vi "Gyro Turn.vi"(6 "degrees":dbl, 9 "If right":bool, 10 "GyroDevRef":T7 {"Sample Rate" min=0.25 max=100.0 step=0.25}, 11 "RobotDriveDevRef in":T1) -> (3 "RobotDriveDevRef out":T1)   [LabVIEW 2017]
uses:
  <vilib>/Rock Robotics/WPI/RobotDrive/WPI_RobotDriveDevRef.ctl
  <vilib>/Rock Robotics/WPI/MotorControl/WPI_MotorControlDeviceRef.ctl
  <vilib>/Rock Robotics/WPI/MotorControl/WPI_MotorControlType.ctl
  <vilib>/Rock Robotics/SystemInterfaces/DIO/FPGA_DIOPWMChannel.ctl
  <vilib>/Rock Robotics/WPI/PWM/WPI_PWMDeadband.ctl
  <vilib>/Rock Robotics/SystemInterfaces/DIO/FPGA_DIOChannel.ctl
  <vilib>/Rock Robotics/WPI/Gyro/WPI_GyroDevRef.ctl
  <vilib>/Rock Robotics/SystemInterfaces/AI/FPGA_AIChannel.ctl
  <vilib>/Rock Robotics/SystemInterfaces/spilib/spi_bus.ctl
  <vilib>/Rock Robotics/WPI/SafetyOutput/WPI_SafetyOutputConfigMenu.ctl
panel:
  # "Analog"
  # "XRS"
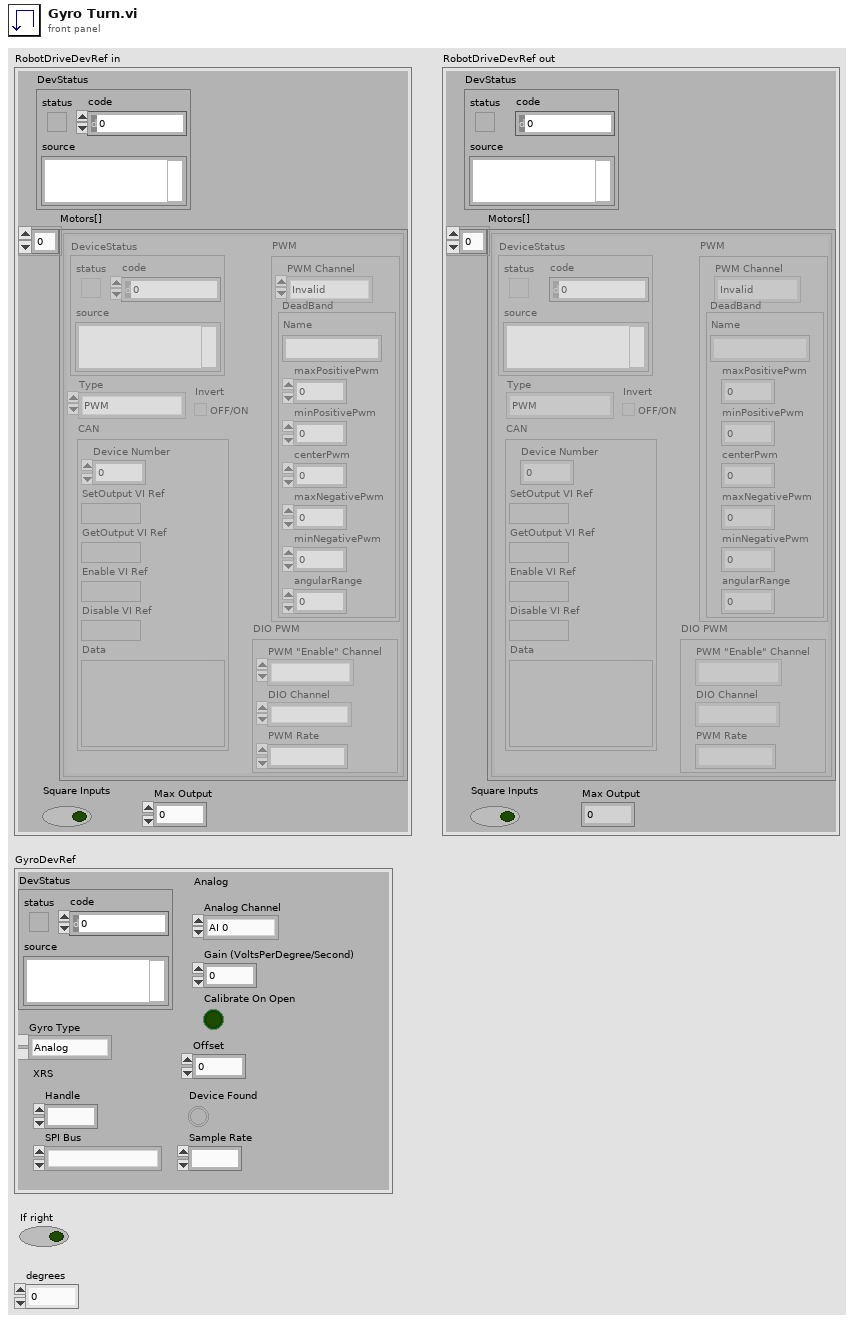
[diagram p1: front panel]
types:
  T1 = typedef "WPI_RobotDriveDevRef.ctl" = cluster{"DevStatus":errorcluster, "Motors[]":T2[], "Square Inputs":bool, "Max Output":dbl}
  T2 = typedef "WPI_MotorControlDeviceRef.ctl" = cluster{"DeviceStatus":errorcluster, "Type":T3, "PWM":cluster{"PWM Channel":T4, "DeadBand":T5}, "CAN":cluster{"Device Number":u8, "SetOutput VI Ref":variant, "GetOutput VI Ref":variant, "Enable VI Ref":variant, "Disable VI Ref":variant, "Data":variant}, "Invert":bool, "DIO PWM":cluster{"PWM \"Enable\" Channel":T4, "DIOChannel":T6, "PWM Rate":dbl}}
  T3 = typedef "WPI_MotorControlType.ctl" = enum16{"PWM", "CAN", "DIO PWM"}
  T4 = typedef "FPGA_DIOPWMChannel.ctl" = enum8{"PWM 0", "PWM 1", "PWM 2", "PWM 3", "PWM 4", "PWM 5", "PWM 6", "PWM 7", "PWM 8", "PWM 9", "PWM MXP 0", "PWM MXP 1", "PWM MXP 2", "PWM MXP 3", "PWM MXP 4", "PWM MXP 5", "PWM MXP 6", "PWM MXP 7", "PWM MXP 8", "PWM MXP 9", "Invalid"}
  T5 = typedef "WPI_PWMDeadband.ctl" = cluster{"Name":string, "maxPositivePwm":i32, "minPositivePwm":i32, "centerPwm":i32, "maxNegativePwm":i32, "minNegativePwm":i32, "angularRange":u16}
  T6 = typedef "FPGA_DIOChannel.ctl" = enum8{"DIO 0", "DIO 1", "DIO 2", "DIO 3", "DIO 4", "DIO 5", "DIO 6", "DIO 7", "DIO 8", "DIO 9", "DIO MXP 0", "DIO MXP 1", "DIO MXP 2", "DIO MXP 3", "DIO MXP 4", "DIO MXP 5", "DIO MXP 6", "DIO MXP 7", "DIO MXP 8", "DIO MXP 9", "DIO MXP 10", "DIO MXP 11", "DIO MXP 12", "DIO MXP 13", "DIO MXP 14", "DIO MXP 15", "SPI Port CS1", "SPI Port CS2", "SPI Port CS3", "SPI Port MISO", "SPI Port MOSI", "Invalid"}
  T7 = typedef "WPI_GyroDevRef.ctl" = cluster{"DevStatus":errorcluster, "Analog Channel":T8, "Gain (VoltsPerDegree/Second)":dbl, "Gyro Type":enum16{"Analog", "XRS450"}, "Handle":i32, "SPI Bus":T9, "Device Found":bool, "Sample Rate":dbl, "Calibrate On Open":bool, "Offset":dbl}
  T8 = typedef "FPGA_AIChannel.ctl" = enum8{"AI 0", "AI 1", "AI 2", "AI 3", "AI MXP 0", "AI MXP 1", "AI MXP 2", "AI MXP 3", "Invalid"}
  T9 = typedef "spi_bus.ctl" = enum16{"SPI On-Board, CS0", "SPI On-Board, CS1", "SPI On-Board, CS2", "SPI On-Board, CS3", "SPI MXP", "Invalid"}
  T10 = typedef "WPI_SafetyOutputConfigMenu.ctl" = enum16{"Enable", "Disable"}
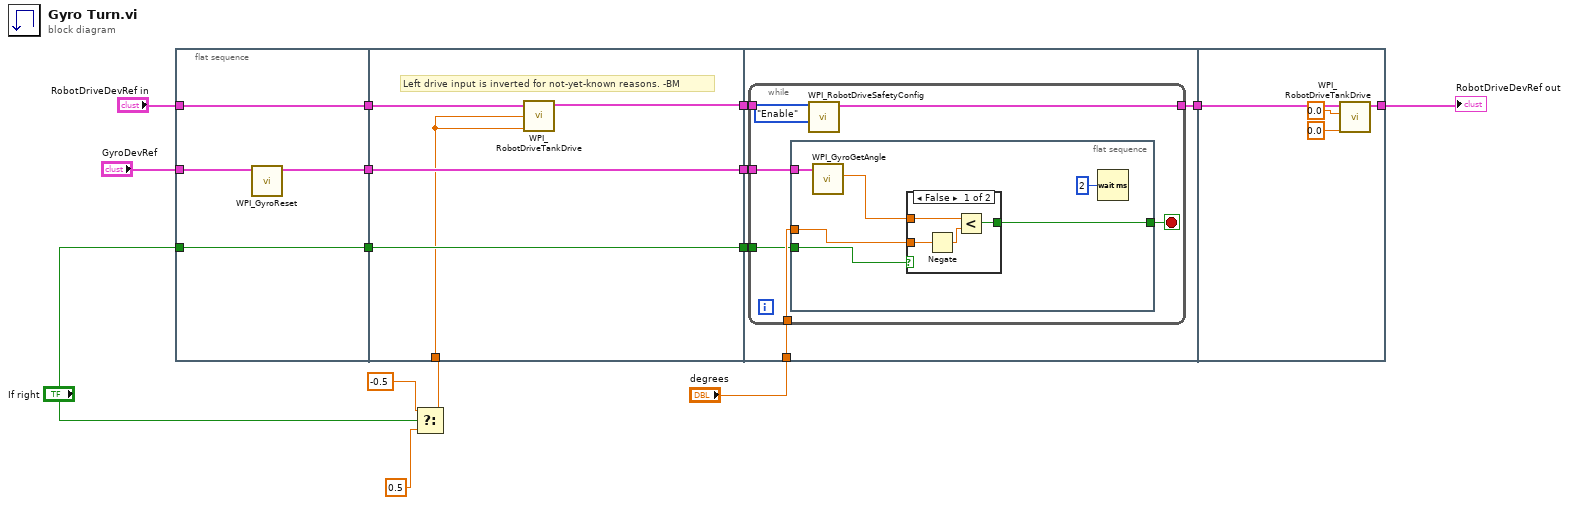
[diagram p0: block diagram]
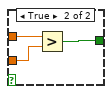
[diagram p2: hidden frame]
diagram:
  n1 = flat-sequence {
    tunnel: "GyroDevRef" -> [w18]
    tunnel: "RobotDriveDevRef in" -> [w19]
    tunnel: [w19] -> w15
    tunnel: [w17] -> w14
    tunnel: "If right" -> [w16]
    tunnel: [w16] -> w2
    tunnel: [w22] -> w13
    tunnel: [w24] -> w12
    tunnel: w15 -> [w23]
    tunnel: w14 -> [w24]
    tunnel: w9 -> [w20]
    tunnel: w2 -> [w21]
    tunnel: [w21] -> w1
    tunnel: "degrees" -> [w27]
    tunnel: [w26] -> w11
    tunnel: w13 -> [w29]
    tunnel: w12 -> [w28]
    tunnel: w1 -> [w25]
    tunnel: w11 -> [w51]
    tunnel: [w50] -> w10
    frame #0 {
      n2 = call <vilib>:"WPI_GyroReset.vi"("GyroDevRef"=w18) -> ("GyroDevRef"=w17:T7)  [unwired: 9 in, 1 out]
    }
    frame #1 {
      # "Left drive input is inverted for not-yet-known reasons. -BM"
      n3 = call <vilib>:"WPI_RobotDriveTankDrive.vi"("Right axis value"=w20, "Left axis value"=w20, "RobotDriveDevRef"=w23) -> ("RobotDriveDevRef"=w22:T1)  [unwired: 6 in, 2 out]
    }
    frame #2 {
      n4 = while {
        tunnel: w29 -> [w36]
        tunnel: w28 -> [w35]
        tunnel: w27 -> [w33]
        tunnel: [w32] -> w26
        tunnel: w25 -> [w31]
        stop <- w34 stop-if-true
        n5 = flat-sequence {
          tunnel: w35 -> [w42]
          tunnel: w33 -> [w40]
          tunnel: [w39] -> w34
          tunnel: w31 -> [w37]
          frame #0 {
            n6 = call <vilib>:"WPI_GyroGetAngle.vi"("GyroDevRef"=w42) -> ("Angle"=w41:dbl)  [unwired: 6 in, 4 out]
            n7 = case shown="False" w37 {
              tunnel: w41 -> [w45 w49]
              tunnel: w40 -> [w44 w48]
              tunnel: [w46 w47] -> w39
              frame False {
                n8 = Negate(x=w44) -> (-x=w43:dbl)
                n9 = Less?(x=w45, y=w43) -> (x < y?=w46:bool)
              }
              frame True {
                n10 = Greater?(x=w49, y=w48) -> (0:w47:bool)
              }
            }
            n11 = Wait (ms)(milliseconds to wait=u32 2) -> ()  [unwired: 1 out]
          }
        }
        n12 = call <vilib>:"WPI_RobotDriveSafetyConfig.vi"("mode"=WPI_SafetyOutputConfigMenu."Enable", "RobotDriveDevRef"=w36) -> ("RobotDriveDevRef"=w32:T1)  [unwired: 8 in, 1 out]
      }
    }
    frame #3 {
      n13 = call <vilib>:"WPI_RobotDriveTankDrive.vi"("Right axis value"=0.0, "Left axis value"=0.0, "RobotDriveDevRef"=w51) -> ("RobotDriveDevRef"=w50:T1)  [unwired: 6 in, 2 out]
    }
  }
  n14 = Select(t=-0.5, s="If right", f=0.5) -> (s? t:f=w9:dbl)
  "RobotDriveDevRef out" <- w10
